vi "Toolkit - Alphabetize Cluster Control.vi"() -> ()   [LabVIEW 2017]
doc: "Alphabetizes a cluster control using VI scripting and the ACE toolkit VIs"
uses:
  <vilib>/Utility/traverseref.llb/TRef TravTarget.ctl
  <vilib>/Utility/traverseref.llb/VI Scripting - Traverse.lvlib
  Toolkit/Toolkit.lvlib
panel:
  out "Change?":bool
  # "Overview: Demonstrates alphabetizing a cluster control using VI scripting the ACE toolkit\nInstructions:\n1. Run this VI\n2. Observe the contents of the cluster control in the target VI that is displayed\n\nThis VI will open the \"Toolkit - Alphabetize Cluster Control Target\" VI, display the front panel before and after alphabetizing of the cluster control in the target VI and then undo the modifications before completing."
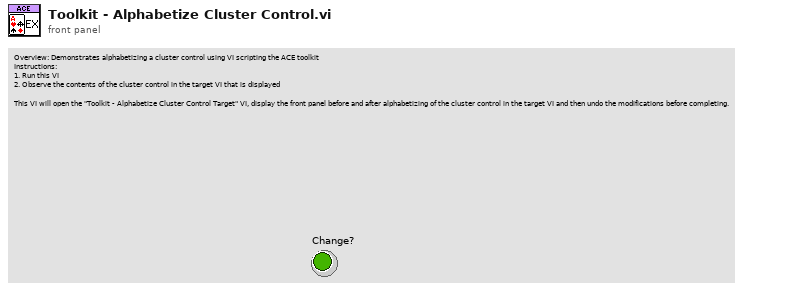
[diagram p1: front panel]
types:
  T1 = enum32{"Invalid", "Standard", "Closed", "Hidden", "Minimized", "Maximized"}
  T2 = typedef "TRef TravTarget.ctl" = enum16{"FP", "BD", "Other"}
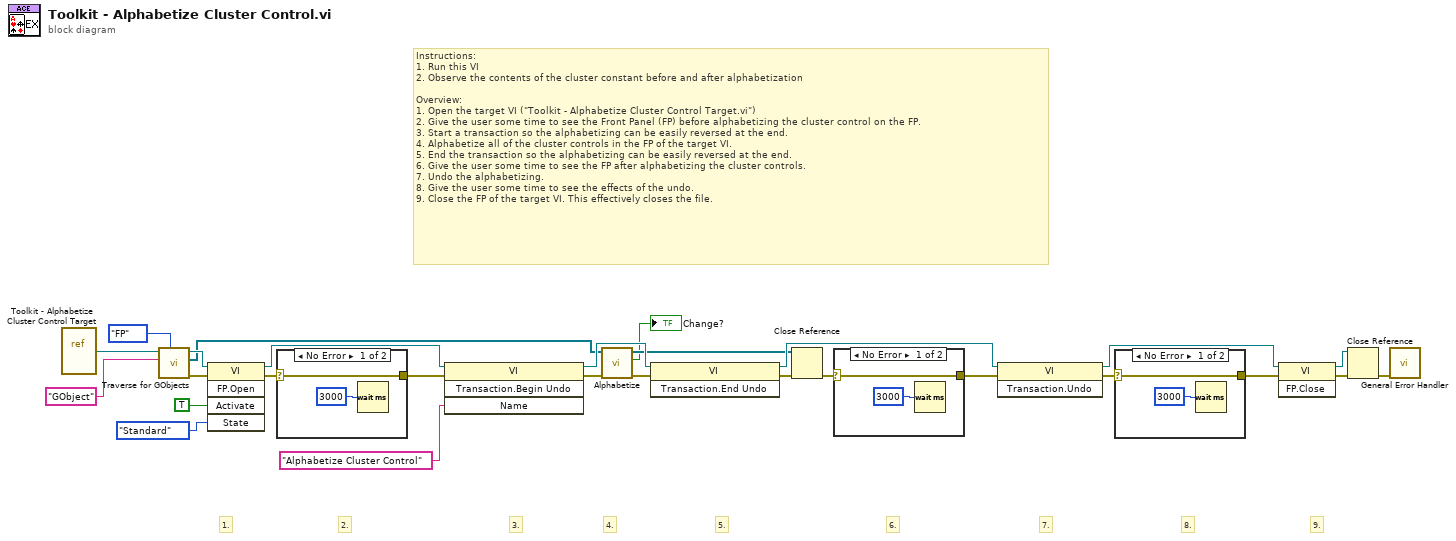
[diagram p0: block diagram]
diagram:
  # "9."
  # "8."
  # "7."
  # "6."
  # "5."
  # "4."
  # "3."
  # "2."
  # "1."
  # "Instructions:\n1. Run this VI\n2. Observe the contents of the cluster constant before and after alphabetization\n\nOverview:\n1. Open the target VI (\"Toolkit - Alphabetize Cluster Control Target.vi\")\n2. Give the user some time to see the Front Panel (FP) before alphabetizing the cluster control on the FP.\n3. Start a transaction so the alphabetizing can be easily reversed at the end.\n4. Alphabetize all of the cluster controls in the FP of the target VI.\n5. End the transaction so the alphabetizing can be easily reversed at the end.\n6. Give the user some time to see the FP after alphabetizing the cluster controls.\n7. Undo the alphabetizing.\n8. Give the user some time to see the effects of the undo.\n9. Close the FP of the target VI. This effectively closes the file."
  n1 = vi-ref "Toolkit - Alphabetize Cluster Control Target.vi"() -> (w3:refnum<vi>)
  n2 = call <vilib>:"Traverse for GObjects.vi"("Traverse Target"=TRef_TravTarget."FP", "Class Name"="GObject", "VI Refnum"=w3) -> ("error out"=w22:errorcluster, "References"=w8:refnum<vi>[], "dup VI Refnum"=w21:refnum<vi>)  [unwired: 5 in, 1 out]
  n3 = invoke class="VI" method="FP.Open"(reference=w21, error in=w22, "Activate"=TRUE ("Activate?"), "State"=T1."Standard") -> (reference out=w20:refnum<vi>, error out=w19:errorcluster)  [unwired: 1 in, 3 out]
  n4 = case shown="No Error" w19 {
    selector: w19 -> [w29 w30]
    tunnel: [w29 w30] -> w16
    frame No Error {
      n5 = Wait (ms)(milliseconds to wait=u32 3000) -> ()  [unwired: 1 out]
    }
    frame Error {
    }
  }
  n6 = invoke class="VI" method="Transaction.Begin Undo"(reference=w20, error in=w16, "Name"="Alphabetize Cluster Control") -> (reference out=w14:refnum<vi>, error out=w4:errorcluster)  [unwired: 1 in, 2 out]
  n7 = call "Alphabetize.vi"("Error In"=w4, "Clusters In"=w8) -> ("Error Out"=w5:errorcluster, "Change?"=→"Change?":bool, "Clusters Out"=w7:refnum<vi>[])  [unwired: 7 in]
  n8 = invoke class="VI" method="Transaction.End Undo"(reference=w14, error in=w5) -> (reference out=w12:refnum<vi>, error out=w13:errorcluster)  [unwired: 1 in, 1 out]
  n9 = Close Reference(reference=w7, error in (no error)=w13) -> (error out=w18:errorcluster)
  n10 = case shown="No Error" w18 {
    selector: w18 -> [w32 w33]
    tunnel: [w32 w33] -> w17
    frame No Error {
      n11 = Wait (ms)(milliseconds to wait=u32 3000) -> ()  [unwired: 1 out]
    }
    frame Error {
    }
  }
  n12 = invoke class="VI" method="Transaction.Undo"(reference=w12, error in=w17) -> (reference out=w11:refnum<vi>, error out=w2:errorcluster)  [unwired: 1 in, 1 out]
  n13 = case shown="No Error" w2 {
    selector: w2 -> [w35 w36]
    tunnel: [w35 w36] -> w1
    frame No Error {
      n14 = Wait (ms)(milliseconds to wait=u32 3000) -> ()  [unwired: 1 out]
    }
    frame Error {
    }
  }
  n15 = invoke class="VI" method="FP.Close"(reference=w11, error in=w1) -> (reference out=w10:refnum<vi>, error out=w9:errorcluster)  [unwired: 1 in, 1 out]
  n16 = Close Reference(reference=w10, error in (no error)=w9) -> (error out=w25:errorcluster)
  n17 = call <vilib>:"General Error Handler.vi"("error in (no error)"=w25) -> ()  [unwired: 10 in, 5 out]
